vi "Pit Scouting.vi"() -> ()   [LabVIEW 2015]
uses:
  <vilib>/Utility/sysdir.llb/System Directory Type.ctl
panel:
  in  "What kind of gearbox?":string
  in  "What does it do?":string
  in  "Vision?":bool
  in  "Low Bar":bool
  in  "Portcullis":bool
  in  "Rough Terrain":bool
  in  "Rock Wall":bool
  in  "Chival de Frise":bool
  in  "Drawbridge":bool
  in  "Sally Port":bool
  in  "Ramparts":bool
  in  "Moat":bool
  in  "Wheel Size":string
  in  "Type of Wheels":string
  in  "Number of Cims?":string
  in  "stop":bool
  in  "What Kind of Robot do they consider themselves?":string(combo)
  in  "Can they scale the tower?":string(combo)
  in  "Team Number":string
  in  "Best attribute about their robot?":string
  in  "High Goal, Low Goal, or Both?":string
  in  "Do they have an Autonomous and what does it do?":string
  in  "What Kind of Drive Train?":string
  # "Obstacles that can be overcome"
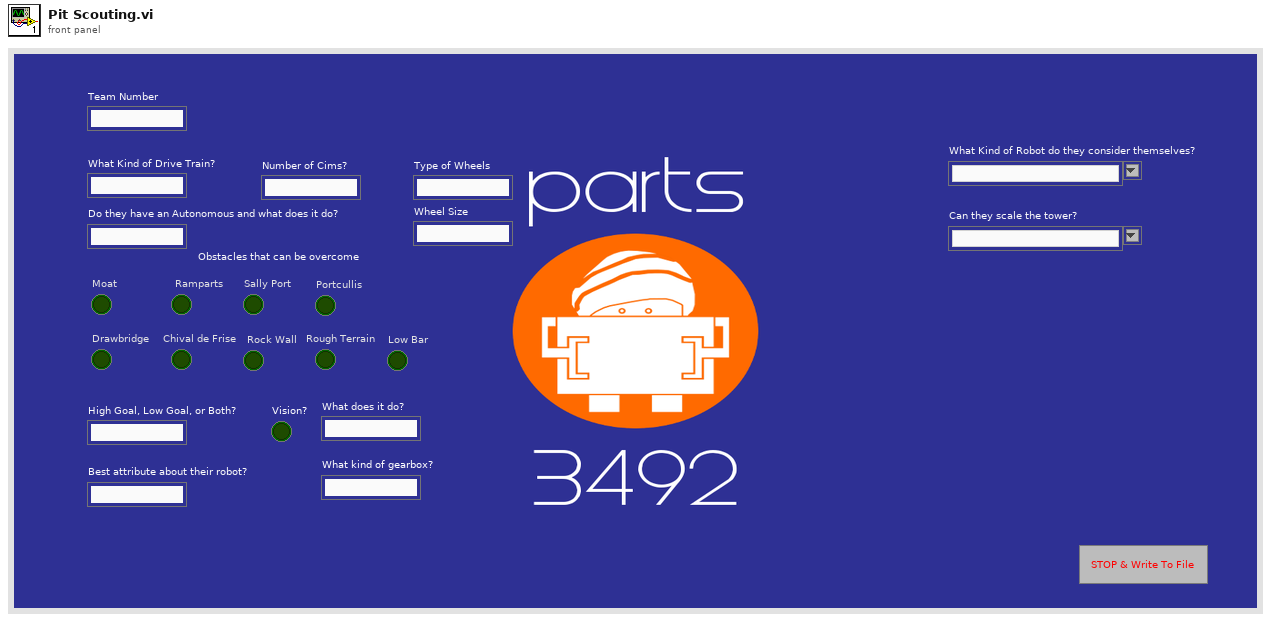
[diagram p1: front panel]
types:
  T1 = typedef "System Directory Type.ctl" = i32
  T2 = enum16{"open", "replace", "create", "open or create", "replace or create", "replace or create with confirmation"}
  T3 = enum32{"invalid app kind", "Development System", "Run Time System", "Student Edition", "Embedded LabVIEW", "Evaluation", "Custom"}
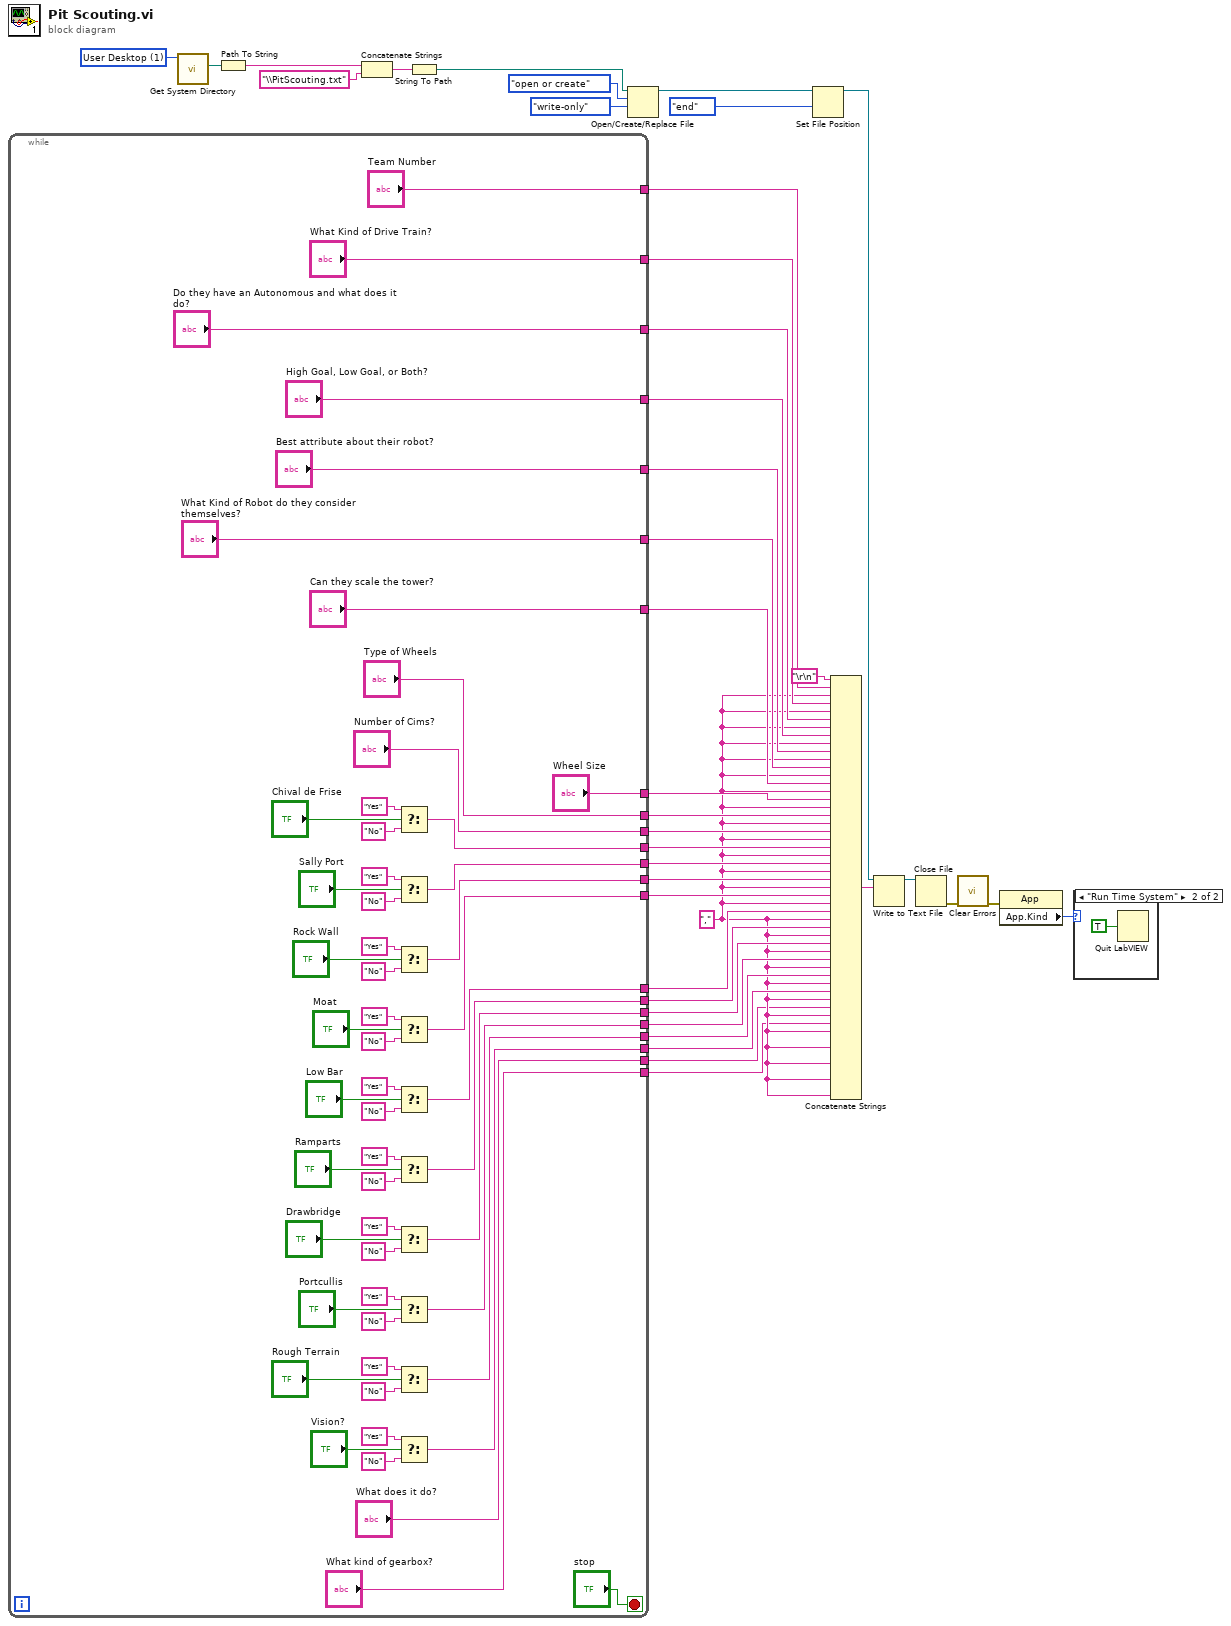
[diagram p0: block diagram]
diagram:
  w35 = T1 1 items=["User Home"=0, "User Desktop"=1, "User Documents"=2, "User Application Data"=3, "User Preferences"=4, "User Temporary"=5, "Public Documents"=6, "Public Application Data"=7, "Public Preferences"=8, "Public Cache"=13, "System Core Libraries"=9, "System Installed Libraries"=10, "Application Files"=11, "Boot Volume Root"=12] ("system directory type")
  w3 = "," ("string")
  n1 = while {
    tunnel: ["Team Number"] -> w23
    tunnel: ["What Kind of Drive Train?"] -> w22
    tunnel: ["Do they have an Autonomous and what does it do?"] -> w21
    tunnel: ["High Goal, Low Goal, or Both?"] -> w20
    tunnel: ["Best attribute about their robot?"] -> w19
    tunnel: ["What Kind of Robot do they consider themselves?"] -> w18
    tunnel: ["Can they scale the tower?"] -> w17
    tunnel: ["Wheel Size"] -> w16
    tunnel: ["Type of Wheels"] -> w15
    tunnel: ["Number of Cims?"] -> w14
    tunnel: [w55] -> w13
    tunnel: [w54] -> w12
    tunnel: [w53] -> w11
    tunnel: [w52] -> w10
    tunnel: [w51] -> w9
    tunnel: [w50] -> w8
    tunnel: [w49] -> w7
    tunnel: [w48] -> w6
    tunnel: [w47] -> w5
    tunnel: [w43] -> w4
    tunnel: ["What does it do?"] -> w2
    tunnel: ["What kind of gearbox?"] -> w1
    stop <- "stop" stop-if-true
    n2 = Select(t="Yes", s="Chival de Frise", f="No") -> (s? t:f=w55:string)
    n3 = Select(t="Yes", s="Sally Port", f="No") -> (s? t:f=w54:string)
    n4 = Select(t="Yes", s="Rock Wall", f="No") -> (s? t:f=w53:string)
    n5 = Select(t="Yes", s="Moat", f="No") -> (s? t:f=w52:string)
    n6 = Select(t="Yes", s="Low Bar", f="No") -> (s? t:f=w51:string)
    n7 = Select(t="Yes", s="Ramparts", f="No") -> (s? t:f=w50:string)
    n8 = Select(t="Yes", s="Drawbridge", f="No") -> (s? t:f=w49:string)
    n9 = Select(t="Yes", s="Portcullis", f="No") -> (s? t:f=w48:string)
    n10 = Select(t="Yes", s="Rough Terrain", f="No") -> (s? t:f=w47:string)
    n11 = Select(t="Yes", s="Vision?", f="No") -> (s? t:f=w43:string)
  }
  n12 = call <vilib>:"Get System Directory.vi"("system directory type"=w35) -> ("system directory"=w34:path)  [unwired: 10 in]
  n13 = Path To String(path=w34) -> (string=w33:string)
  n14 = Concatenate Strings(w33, "\\PitScouting.txt" ("string")) -> (w31:string)
  n15 = String To Path(string=w31) -> (path=w30:path)
  n16 = Open/Create/Replace File(file path (use dialog)=w30, operation (0:open)=T2."open or create", access (0:read/write)=enum16{"read/write", "read-only", "write-only"}."write-only") -> (refnum out=w37:refnum<file>)  [unwired: 3 in, 2 out]
  n17 = Set File Position(refnum=w37, from (0:start)=enum16{"start", "end", "current"}."end") -> (refnum out=w25:refnum<file>)  [unwired: 2 in, 1 out]
  n18 = Concatenate Strings("\r\n", w23, w3, w22, w3, w21, w3, w20, w3, w19, w3, w18, w3, w17, w3, w16, w3, w15, w3, w14, w3, w13, w3, w12, w3, w11, w3, w10, w3, w9, w3, w8, w3, w7, w3, w6, w3, w5, w3, w4, w3, w2, w3, w1, w3, w3, w3, w3, w3) -> (w24:string)  [unwired: 4 in]
  n19 = Write to Text File(file (use dialog)=w25, text=w24) -> (refnum out=w29:refnum<file>)  [unwired: 2 in, 2 out]
  n20 = Close File(refnum=w29) -> (error out=w28:errorcluster)  [unwired: 1 in, 1 out]
  n21 = call <vilib>:"Clear Errors.vi"("error in (no error)"=w28) -> ("error out"=w27:errorcluster)  [unwired: 5 in, 1 out]
  n22 = property class="App"(error in=w27) -> ("App.Kind"=w26:T3)  [unwired: 1 in, 2 out]
  n23 = case shown="\"Run Time System\"" w26 {
    frame Default {
    }
    frame "Run Time System" {
      n24 = Quit LabVIEW(quit? (T)=TRUE) -> ()
    }
  }
